vi "CH_LM App DAQ Stop.vi"(4 "error in (no error)":errorcluster, 6 "rendezvous":T3, 7 "i ref":refnum<vi>) -> (0 "error out":errorcluster, 2 "timed out":bool, 3 "i ref":refnum<vi>)   [LabVIEW 2012, in "CH_LM App.lvlib"]
doc: "This VI can be used to stop the DAQ thread."
uses:
  CH_LM App.lvlib
  CH_LM App DAQ Command.ctl
  CH_LM/CH_LM Measurement Delivery Mode.ctl
  CH_LM.lvlib
panel:
  in  "DAQ Command":T1={"Wait at Rendesvouz"=FALSE, "Command"="", "Sample Collection"=enum."Continuous", "Sample Size"=100, "Collection Mode"=enum."Streaming", "T / ms"=1.0, "NofBins"=7, "Point(s)"=1, "Log Data File"=path "", "Log data to File"=FALSE, "Pause"=FALSE, "Meter Index"=0, "Data format"=0, "Delivery Mode"=enum."Last", "Start/Stop Button"=refnum, "Point(s) Array"=[]} {"Point(s) Array" min=1 max=20000; "Point(s)" min=1 max=20000; "Sample Size" min=1}
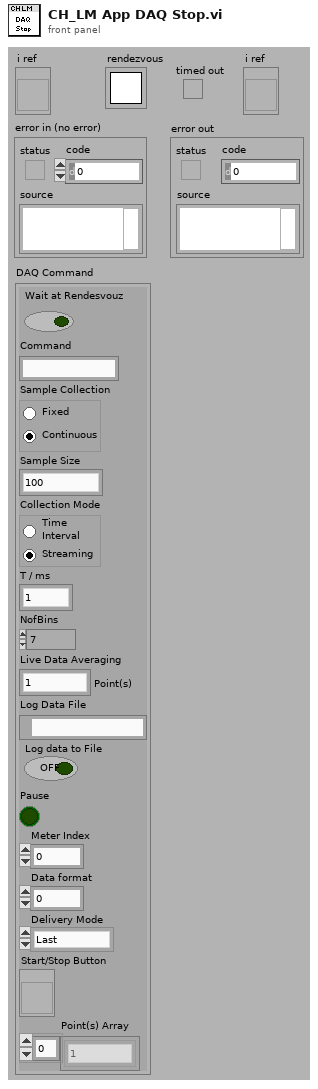
[diagram p1: front panel]
types:
  T1 = typedef "CH_LM App.lvlib/CH_LM App DAQ Command.ctl" = cluster{"Wait at Rendesvouz":bool, "Command":string, "Sample Collection":enum32{"Fixed", "Continuous"}, "Sample Size":i32, "Collection Mode":enum32{"Time\nInterval", "Streaming"}, "T / ms":dbl, "NofBins":i32, "Point(s)":u32, "Log Data File":path, "Log data to File":bool, "Pause":bool, "Meter Index":i32, "Data format":u16, "Delivery Mode":T2, "Start/Stop Button":refnum<vi>, "Point(s) Array":u32[]}
  T2 = typedef "CH_LM.lvlib/CH_LM Measurement Delivery Mode.ctl" = enum16{"Last", "Stream"}
  T3 = typedef "Rendezvous RefNum" = refnum<k1>
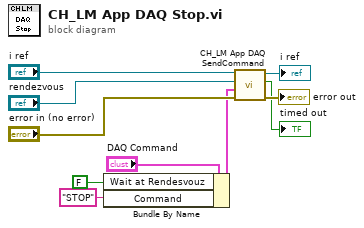
[diagram p0: block diagram]
diagram:
  n1 = Bundle By Name(cluster="DAQ Command", "Wait at Rendesvouz"=FALSE, "Command"="STOP") -> (w2:T1)
  n2 = call "CH_LM App DAQ SendCommand.vi"("error in (no error)"="error in (no error)", "DAQ Command"=w2, "rendezvous"="rendezvous", "i ref"="i ref") -> ("error out"=→"error out":errorcluster, "timed out"=→"timed out":bool, "i ref"=→"i ref":refnum<vi>)  [unwired: 1 out]
